vi "test_Restart.vi"() -> ()   [LabVIEW 2020]
panel:
  out "iterations":i32
  in  "milliseconds to wait":u32
  in  "stop":bool
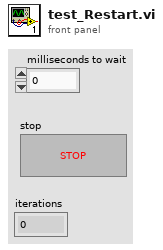
[diagram p1: front panel]
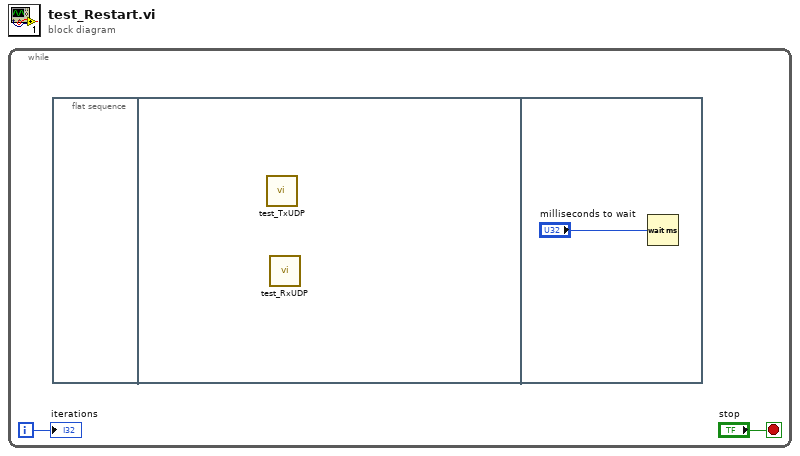
[diagram p0: block diagram]
diagram:
  n1 = while {
    i -> [w1]
    stop <- "stop" stop-if-true
    n2 = flat-sequence {
      frame #0 {
      }
      frame #1 {
        n3 = call "test_TxUDP.vi"() -> ()  [unwired: 12 in]
        n4 = call "test_RxUDP.vi"() -> ()  [unwired: 12 in]
      }
      frame #2 {
        n5 = Wait (ms)(milliseconds to wait="milliseconds to wait") -> ()  [unwired: 1 out]
      }
    }
    "iterations" <- w1
  }
